vi "unregisterSubscriber.vi"(1 "Parameters":T3) -> (2 "Error out":errorcluster, 3 "Reply":T2, 4 "Log":T1)   [LabVIEW 2012]
uses:
  _ROSDefinition.vi
  Console/Servers/ServerSubs/ROSLog.ctl
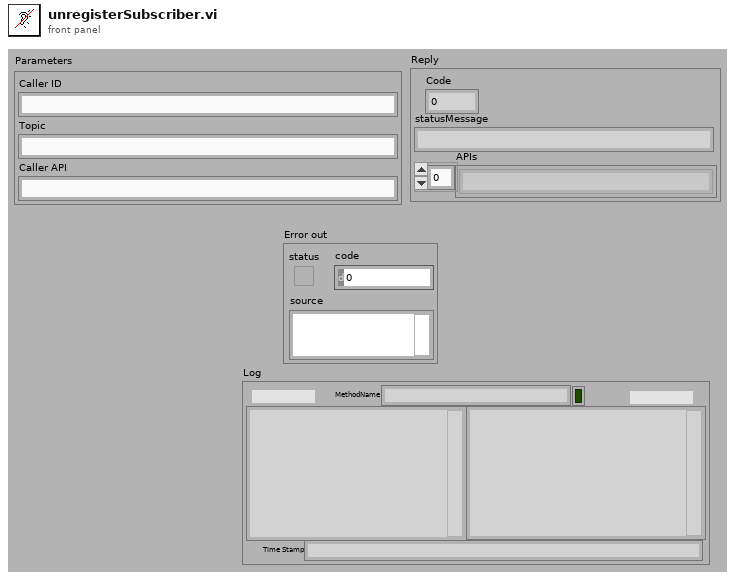
[diagram p1: front panel]
types:
  T1 = typedef "ROSLog.ctl" = cluster{"Sent":string, "Reply":string, "MethodName":string, "success":bool, "Dir1":string, "Dir2":string, "Time Stamp":string}
  T2 = cluster{"Code":i8, "statusMessage":string, "APIs":string[]}
  T3 = cluster{"Caller ID":string, "Topic":string, "Caller API":string}
  T4 = cluster{"Code":i8, "statusMessage":string, "APIs":string[]}[]
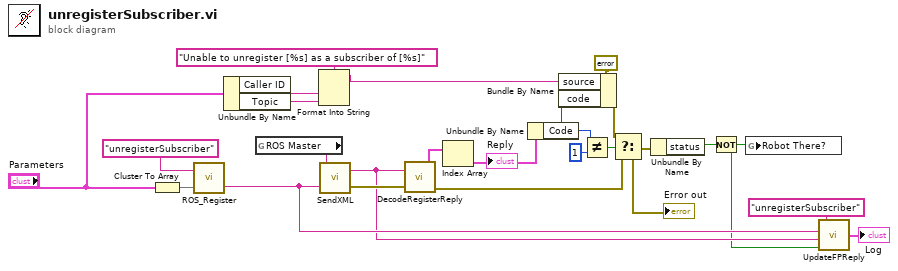
[diagram p0: block diagram]
diagram:
  n1 = Cluster To Array(cluster="Parameters") -> (array=w7:string[])
  n2 = call "ROS_Register.vi"("Parameters"=w7, "Method Name"="unregisterSubscriber") -> ("registerSubscriber"=w5:string)  [unwired: 1 in]
  n3 = Unbundle By Name("Parameters") -> ("Caller ID"=w22:string, "Topic"=w21:string)
  n4 = global read "_ROSDefinition.vi" "ROS Master"() -> (w24:string)
  n5 = Format Into String(format string="Unable to unregister [%s] as a subscriber of [%s]" ("source"), w22, w21) -> (resulting string=w10:string)  [unwired: 2 in, 1 out]
  n6 = call "SendXML.vi"("Send"=w5, "URI in"=w24) -> ("error out"=w11:errorcluster, "Reply"=w4:string)
  n7 = call "DecodeRegisterReply.vi"("error in (no error)"=w11, "Response"=w4) -> ("error out"=w15:errorcluster, "Reply"=w19:T4)
  n8 = Index Array(array=w19) -> (element=w18:T2)  [unwired: 1 in]
  "Reply" <- w18
  n9 = Unbundle By Name(w18) -> ("Code"=w14:i8)
  n10 = Bundle By Name(cluster=errorcluster {"status"=TRUE, "code"=0, "source"=" Error"} ("t"), "source"=w10, "code"=w14) -> (w13:errorcluster)
  n11 = Not Equal?(x=w14, y=i8 1) -> (x != y?=w16:bool)
  n12 = Select(t=w13, s=w16, f=w15) -> (s? t:f=w12:errorcluster)
  "Error out" <- w12
  n13 = Unbundle By Name(w12) -> ("status"=w20:bool)
  n14 = Not(x=w20) -> (.not. x?=w2:bool)
  n15 = global write "_ROSDefinition.vi" "Robot There?"(w2) -> ()
  n16 = call "UpdateFPReply.vi"("success?"=w2, "Reply"=w4, "Sent"=w5, "method"="unregisterSubscriber" ("name (unnamed)")) -> ("Log"=→"Log":T1)
